vi "Cypher Driver.vi"() -> ()   [LabVIEW 2016]
uses:
  <userlib>/LevyLab/Relay Box/Type_defs/Resistor--enum.ctl
  subVIs/Driver Variables_Cypher.vi
  subVIs/Global Variables.vi
panel:
  in  "Data Queue":refnum<queue>
  in  "Amplifier Setting":dbl=-15.0
  in  "Interpolation Distance (µm)":dbl=0.1
  in  "Background Image":refnum<vi>
  in  "Inkscape File (.svg)":refnum<vi>
  in  "Run":refnum<vi>
  in  "Abort":refnum<vi>
  in  "Lithography Data":T2(array[cluster])=[{"Name"="f0", "Litho"=[{"X"=29.513355999999998, "Y"=9.417726199999999, "Speed"=5.0, "Voltage"=12.0}, {"X"=29.178072445529672, "Y"=9.536088907738542, "Speed"=5.0, "Voltage"=12.0}, {"X"=28.835439481592786, "Y"=9.643840890007512, "Speed"=5.0, "Voltage"=12.0}, {"X"=28.47974138467318, "Y"=9.7371182081142, "Speed"=5.0, "Voltage"=12.0}, {"X"=28.105262431254694, "Y"=9.812056923365887, "Speed"=5.0, "Voltage"=12.0}, {"X"=27.706286897821187, "Y"=9.864793097069871, "Speed"=5.0, "Voltage"=12.0}, {"X"=27.277099060856493, "Y"=9.891462790533431, "Speed"=5.0, "Voltage"=12.0}, {"X"=26.811983196844476, "Y"=9.88820206506386, "Speed"=5.0, "Voltage"=12.0}, {"X"=26.305223582268965, "Y"=9.851146981968443, "Speed"=5.0, "Voltage"=12.0}, {"X"=25.751104493613816, "Y"=9.776433602554466, "Speed"=5.0, "Voltage"=12.0}, {"X"=25.14391020736288, "Y"=9.660197988129223, "Speed"=5.0, "Voltage"=12.0}, {"X"=24.477925, "Y"=9.498576199999999, "Speed"=5.0, "Voltage"=12.0}, {"X"=24.477925, "Y"=9.498576199999999, "Speed"=5.0, "Voltage"=12.0}, {"X"=25.11834108313298, "Y"=9.668960284590531, "Speed"=5.0, "Voltage"=12.0}, {"X"=25.70468663448534, "Y"=9.797549343831701, "Speed"=5.0, "Voltage"=12.0}, {"X"=26.242539884259948, "Y"=9.887743940473326, "Speed"=5.0, "Voltage"=12.0}, {"X"=26.737479062659652, "Y"=9.942944637265212, "Speed"=5.0, "Voltage"=12.0}, {"X"=27.195082399887298, "Y"=9.966551996957172, "Speed"=5.0, "Voltage"=12.0}, {"X"=27.620928126145756, "Y"=9.961966582299022, "Speed"=5.0, "Voltage"=12.0}, {"X"=28.020594471637867, "Y"=9.932588956040568, "Speed"=5.0, "Voltage"=12.0}, {"X"=28.399659666566492, "Y"=9.881819680931631, "Speed"=5.0, "Voltage"=12.0}, {"X"=28.763701941134485, "Y"=9.813059319722012, "Speed"=5.0, "Voltage"=12.0}, {"X"=29.1182995255447, "Y"=9.729708435161532, "Speed"=5.0, "Voltage"=12.0}, {"X"=29.469030649999997, "Y"=9.635167589999998, "Speed"=5.0, "Voltage"=12.0}, {"X"=29.4247053, "Y"=9.85260898, "Speed"=5.0, "Voltage"=12.0}, {"X"=29.058526605559724, "Y"=9.923327962584523, "Speed"=5.0, "Voltage"=12.0}, {"X"=28.69196440067618, "Y"=9.982277749436513, "Speed"=5.0, "Voltage"=12.0}, {"X"=28.319577948459806, "Y"=10.02652115374906, "Speed"=5.0, "Voltage"=12.0}, {"X"=27.935926512021034, "Y"=10.053120988715248, "Speed"=5.0, "Voltage"=12.0}, {"X"=27.535569354470322, "Y"=10.059140067528173, "Speed"=5.0, "Voltage"=12.0}, {"X"=27.113065738918102, "Y"=10.041641203380916, "Speed"=5.0, "Voltage"=12.0}, {"X"=26.662974928474828, "Y"=9.997687209466564, "Speed"=5.0, "Voltage"=12.0}, {"X"=26.179856186250937, "Y"=9.92434089897821, "Speed"=5.0, "Voltage"=12.0}, {"X"=25.658268775356866, "Y"=9.818665085108938, "Speed"=5.0, "Voltage"=12.0}, {"X"=25.092771958903075, "Y"=9.677722581051837, "Speed"=5.0, "Voltage"=12.0}, {"X"=24.477924999999995, "Y"=9.498576199999999, "Speed"=5.0, "Voltage"=12.0}, {"X"=24.477925, "Y"=9.498576199999999, "Speed"=5.0, "Voltage"=12.0}, {"X"=25.067202834673175, "Y"=9.686484877513145, "Speed"=5.0, "Voltage"=12.0}, {"X"=25.61185091622839, "Y"=9.839780826386171, "Speed"=5.0, "Voltage"=12.0}, {"X"=26.11717248824192, "Y"=9.960937857483094, "Speed"=5.0, "Voltage"=12.0}, {"X"=26.588470794290004, "Y"=10.052429781667916, "Speed"=5.0, "Voltage"=12.0}, {"X"=27.031049077948904, "Y"=10.116730409804656, "Speed"=5.0, "Voltage"=12.0}, {"X"=27.45021058279489, "Y"=10.156313552757323, "Speed"=5.0, "Voltage"=12.0}, {"X"=27.851258552404204, "Y"=10.17365302138993, "Speed"=5.0, "Voltage"=12.0}, {"X"=28.23949623035312, "Y"=10.171222626566491, "Speed"=5.0, "Voltage"=12.0}, {"X"=28.62022686021788, "Y"=10.151496179151012, "Speed"=5.0, "Voltage"=12.0}, {"X"=28.99875368557475, "Y"=10.116947490007512, "Speed"=5.0, "Voltage"=12.0}, {"X"=29.38037995, "Y"=10.070050369999997, "Speed"=5.0, "Voltage"=12.0}, {"X"=29.336054599999997, "Y"=10.287491759999998, "Speed"=5.0, "Voltage"=12.0}, {"X"=28.938980765589776, "Y"=10.310567017430502, "Speed"=5.0, "Voltage"=12.0}, {"X"=28.548489319759575, "Y"=10.320714608865513, "Speed"=5.0, "Voltage"=12.0}, {"X"=28.159414512246432, "Y"=10.315924099383922, "Speed"=5.0, "Voltage"=12.0}, {"X"=27.766590592787374, "Y"=10.29418505406461, "Speed"=5.0, "Voltage"=12.0}, {"X"=27.364851811119458, "Y"=10.253487037986474, "Speed"=5.0, "Voltage"=12.0}, {"X"=26.94903241697971, "Y"=10.191819616228399, "Speed"=5.0, "Voltage"=12.0}, {"X"=26.513966660105183, "Y"=10.10717235386927, "Speed"=5.0, "Voltage"=12.0}, {"X"=26.054488790232902, "Y"=9.997534815987978, "Speed"=5.0, "Voltage"=12.0}, {"X"=25.565433057099916, "Y"=9.860896567663406, "Speed"=5.0, "Voltage"=12.0}, {"X"=25.04163371044327, "Y"=9.695247173974453, "Speed"=5.0, "Voltage"=12.0}, {"X"=24.477925, "Y"=9.498576199999999, "Speed"=5.0, "Voltage"=12.0}, {"X"=24.477925, "Y"=9.498576199999999, "Speed"=5.0, "Voltage"=12.0}, {"X"=25.016064586213368, "Y"=9.70400947043576, "Speed"=5.0, "Voltage"=12.0}, {"X"=25.51901519797144, "Y"=9.882012308940642, "Speed"=5.0, "Voltage"=12.0}, {"X"=25.99180509222389, "Y"=10.034131774492861, "Speed"=5.0, "Voltage"=12.0}, {"X"=26.439462525920355, "Y"=10.161914926070622, "Speed"=5.0, "Voltage"=12.0}, {"X"=26.867015756010513, "Y"=10.26690882265214, "Speed"=5.0, "Voltage"=12.0}, {"X"=27.279493039444027, "Y"=10.350660523215627, "Speed"=5.0, "Voltage"=12.0}, {"X"=27.681922633170547, "Y"=10.41471708673929, "Speed"=5.0, "Voltage"=12.0}, {"X"=28.079332794139745, "Y"=10.460625572201351, "Speed"=5.0, "Voltage"=12.0}, {"X"=28.476751779301274, "Y"=10.489933038580013, "Speed"=5.0, "Voltage"=12.0}, {"X"=28.879207845604803, "Y"=10.504186544853493, "Speed"=5.0, "Voltage"=12.0}, {"X"=29.291729249999996, "Y"=10.50493315, "Speed"=5.0, "Voltage"=12.0}, {"X"=29.2474039, "Y"=10.722374539999999, "Speed"=5.0, "Voltage"=12.0}, {"X"=28.81943492561983, "Y"=10.697806072276482, "Speed"=5.0, "Voltage"=12.0}, {"X"=28.405014238842973, "Y"=10.659151468294514, "Speed"=5.0, "Voltage"=12.0}, {"X"=27.999251076033058, "Y"=10.605327045018782, "Speed"=5.0, "Voltage"=12.0}, {"X"=27.597254673553717, "Y"=10.535249119413972, "Speed"=5.0, "Voltage"=12.0}, {"X"=27.194134267768597, "Y"=10.447834008444776, "Speed"=5.0, "Voltage"=12.0}, {"X"=26.784999095041314, "Y"=10.341998029075882, "Speed"=5.0, "Voltage"=12.0}, {"X"=26.364958391735534, "Y"=10.216657498271974, "Speed"=5.0, "Voltage"=12.0}, {"X"=25.92912139421487, "Y"=10.070728732997745, "Speed"=5.0, "Voltage"=12.0}, {"X"=25.472597338842967, "Y"=9.903128050217878, "Speed"=5.0, "Voltage"=12.0}, {"X"=24.99049546198347, "Y"=9.712771766897067, "Speed"=5.0, "Voltage"=12.0}, {"X"=24.477925, "Y"=9.498576199999999, "Speed"=5.0, "Voltage"=12.0}, {"X"=24.477925, "Y"=9.498576199999999, "Speed"=5.0, "Voltage"=12.0}, {"X"=24.964926337753568, "Y"=9.721534063358375, "Speed"=5.0, "Voltage"=12.0}, {"X"=25.42617947971449, "Y"=9.924243791495112, "Speed"=5.0, "Voltage"=12.0}, {"X"=25.866437696205857, "Y"=10.107325691502629, "Speed"=5.0, "Voltage"=12.0}, {"X"=26.29045425755071, "Y"=10.271400070473327, "Speed"=5.0, "Voltage"=12.0}, {"X"=26.70298243407212, "Y"=10.417087235499622, "Speed"=5.0, "Voltage"=12.0}, {"X"=27.108775496093163, "Y"=10.545007493673928, "Speed"=5.0, "Voltage"=12.0}, {"X"=27.512586713936884, "Y"=10.655781152088654, "Speed"=5.0, "Voltage"=12.0}, {"X"=27.91916935792637, "Y"=10.750028517836213, "Speed"=5.0, "Voltage"=12.0}, {"X"=28.333276698384672, "Y"=10.828369898009015, "Speed"=5.0, "Voltage"=12.0}, {"X"=28.759662005634855, "Y"=10.891425599699472, "Speed"=5.0, "Voltage"=12.0}, {"X"=29.203078549999997, "Y"=10.939815929999998, "Speed"=5.0, "Voltage"=12.0}, {"X"=29.1587532, "Y"=11.15725732, "Speed"=5.0, "Voltage"=12.0}, {"X"=28.69988908564988, "Y"=11.085045127122463, "Speed"=5.0, "Voltage"=12.0}, {"X"=28.261539157926368, "Y"=10.997588327723514, "Speed"=5.0, "Voltage"=12.0}, {"X"=27.839087639819684, "Y"=10.894729990653644, "Speed"=5.0, "Voltage"=12.0}, {"X"=27.427918754320057, "Y"=10.776313184763334, "Speed"=5.0, "Voltage"=12.0}, {"X"=27.023416724417732, "Y"=10.642180978903077, "Speed"=5.0, "Voltage"=12.0}, {"X"=26.620965773102924, "Y"=10.492176441923366, "Speed"=5.0, "Voltage"=12.0}, {"X"=26.215950123365886, "Y"=10.326142642674679, "Speed"=5.0, "Voltage"=12.0}, {"X"=25.803753998196843, "Y"=10.143922650007513, "Speed"=5.0, "Voltage"=12.0}, {"X"=25.379761620586017, "Y"=9.945359532772349, "Speed"=5.0, "Voltage"=12.0}, {"X"=24.939357213523664, "Y"=9.730296359819683, "Speed"=5.0, "Voltage"=12.0}, {"X"=24.477925, "Y"=9.498576199999999, "Speed"=5.0, "Voltage"=12.0}, {"X"=24.477925, "Y"=9.498576199999999, "Speed"=5.0, "Voltage"=12.0}, {"X"=24.91378808929376, "Y"=9.739058656280989, "Speed"=5.0, "Voltage"=12.0}, {"X"=25.33334376145754, "Y"=9.966475274049584, "Speed"=5.0, "Voltage"=12.0}, {"X"=25.74107030018783, "Y"=10.180519608512395, "Speed"=5.0, "Voltage"=12.0}, {"X"=26.141445989181065, "Y"=10.38088521487603, "Speed"=5.0, "Voltage"=12.0}, {"X"=26.53894911213373, "Y"=10.567265648347107, "Speed"=5.0, "Voltage"=12.0}, {"X"=26.938057952742298, "Y"=10.73935446413223, "Speed"=5.0, "Voltage"=12.0}, {"X"=27.343250794703227, "Y"=10.896845217438013, "Speed"=5.0, "Voltage"=12.0}, {"X"=27.759005921712998, "Y"=11.039431463471075, "Speed"=5.0, "Voltage"=12.0}, {"X"=28.189801617468063, "Y"=11.166806757438014, "Speed"=5.0, "Voltage"=12.0}, {"X"=28.64011616566491, "Y"=11.278664654545453, "Speed"=5.0, "Voltage"=12.0}, {"X"=29.11442785, "Y"=11.37469871, "Speed"=5.0, "Voltage"=12.0}, {"X"=29.070102499999997, "Y"=11.592140099999998, "Speed"=5.0, "Voltage"=12.0}, {"X"=28.580343245679934, "Y"=11.472284181968444, "Speed"=5.0, "Voltage"=12.0}, {"X"=28.118064077009763, "Y"=11.336025187152515, "Speed"=5.0, "Voltage"=12.0}, {"X"=27.678924203606314, "Y"=11.184132936288504, "Speed"=5.0, "Voltage"=12.0}, {"X"=27.258582835086397, "Y"=11.017377250112695, "Speed"=5.0, "Voltage"=12.0}, {"X"=26.852699181066864, "Y"=10.83652794936138, "Speed"=5.0, "Voltage"=12.0}, {"X"=26.456932451164533, "Y"=10.642354854770847, "Speed"=5.0, "Voltage"=12.0}, {"X"=26.066941854996237, "Y"=10.435627787077383, "Speed"=5.0, "Voltage"=12.0}, {"X"=25.67838660217881, "Y"=10.217116567017278, "Speed"=5.0, "Voltage"=12.0}, {"X"=25.28692590232907, "Y"=9.987591015326819, "Speed"=5.0, "Voltage"=12.0}, {"X"=24.888218965063857, "Y"=9.747820952742297, "Speed"=5.0, "Voltage"=12.0}, {"X"=24.477925, "Y"=9.498576199999999, "Speed"=5.0, "Voltage"=12.0}, {"X"=24.477925, "Y"=9.498576199999999, "Speed"=5.0, "Voltage"=12.0}, {"X"=24.862649840833956, "Y"=9.756583249203604, "Speed"=5.0, "Voltage"=12.0}, {"X"=25.240508043200595, "Y"=10.008706756604054, "Speed"=5.0, "Voltage"=12.0}, {"X"=25.615702904169794, "Y"=10.253713525522164, "Speed"=5.0, "Voltage"=12.0}, {"X"=25.992437720811417, "Y"=10.490370359278735, "Speed"=5.0, "Voltage"=12.0}, {"X"=26.374915790195338, "Y"=10.717444061194591, "Speed"=5.0, "Voltage"=12.0}, {"X"=26.767340409391434, "Y"=10.933701434590532, "Speed"=5.0, "Voltage"=12.0}, {"X"=27.17391487546957, "Y"=11.137909282787376, "Speed"=5.0, "Voltage"=12.0}, {"X"=27.598842485499624, "Y"=11.328834409105935, "Speed"=5.0, "Voltage"=12.0}, {"X"=28.04632653655146, "Y"=11.505243616867016, "Speed"=5.0, "Voltage"=12.0}, {"X"=28.520570325694962, "Y"=11.665903709391433, "Speed"=5.0, "Voltage"=12.0}, {"X"=29.02577715, "Y"=11.80958149, "Speed"=5.0, "Voltage"=12.0}, {"X"=28.981451800000002, "Y"=12.02702288, "Speed"=5.0, "Voltage"=12.0}, {"X"=28.46079740570999, "Y"=11.859523236814423, "Speed"=5.0, "Voltage"=12.0}, {"X"=27.97458899609316, "Y"=11.674462046581516, "Speed"=5.0, "Voltage"=12.0}, {"X"=27.51876076739294, "Y"=11.473535881923366, "Speed"=5.0, "Voltage"=12.0}, {"X"=27.08924691585274, "Y"=11.258441315462056, "Speed"=5.0, "Voltage"=12.0}, {"X"=26.681981637716, "Y"=11.030874919819684, "Speed"=5.0, "Voltage"=12.0}, {"X"=26.292899129226143, "Y"=10.792533267618332, "Speed"=5.0, "Voltage"=12.0}, {"X"=25.917933586626592, "Y"=10.545112931480087, "Speed"=5.0, "Voltage"=12.0}, {"X"=25.55301920616078, "Y"=10.290310484027048, "Speed"=5.0, "Voltage"=12.0}, {"X"=25.19409018407212, "Y"=10.02982249788129, "Speed"=5.0, "Voltage"=12.0}, {"X"=24.837080716604056, "Y"=9.76534554566491, "Speed"=5.0, "Voltage"=12.0}, {"X"=24.477925, "Y"=9.498576199999999, "Speed"=5.0, "Voltage"=12.0}, {"X"=24.477925, "Y"=9.498576199999999, "Speed"=5.0, "Voltage"=12.0}, {"X"=24.811511592374153, "Y"=9.774107842126218, "Speed"=5.0, "Voltage"=12.0}, {"X"=25.147672324943645, "Y"=10.050938239158524, "Speed"=5.0, "Voltage"=12.0}, {"X"=25.490335508151766, "Y"=10.32690744253193, "Speed"=5.0, "Voltage"=12.0}, {"X"=25.843429452441768, "Y"=10.59985550368144, "Speed"=5.0, "Voltage"=12.0}, {"X"=26.210882468256948, "Y"=10.867622474042072, "Speed"=5.0, "Voltage"=12.0}, {"X"=26.59662286604057, "Y"=11.128048405048833, "Speed"=5.0, "Voltage"=12.0}, {"X"=27.00457895623591, "Y"=11.378973348136737, "Speed"=5.0, "Voltage"=12.0}, {"X"=27.43867904928625, "Y"=11.618237354740796, "Speed"=5.0, "Voltage"=12.0}, {"X"=27.902851455634856, "Y"=11.843680476296015, "Speed"=5.0, "Voltage"=12.0}, {"X"=28.401024485725014, "Y"=12.053142764237414, "Speed"=5.0, "Voltage"=12.0}, {"X"=28.93712645, "Y"=12.24446427, "Speed"=5.0, "Voltage"=12.0}, {"X"=28.8928011, "Y"=12.46190566, "Speed"=5.0, "Voltage"=12.0}, {"X"=28.34125156574004, "Y"=12.246762291660403, "Speed"=5.0, "Voltage"=12.0}, {"X"=27.831113915176555, "Y"=12.012898906010516, "Speed"=5.0, "Voltage"=12.0}, {"X"=27.358597331179567, "Y"=11.762938827558227, "Speed"=5.0, "Voltage"=12.0}, {"X"=26.91991099661908, "Y"=11.499505380811417, "Speed"=5.0, "Voltage"=12.0}, {"X"=26.51126409436514, "Y"=11.225221890277984, "Speed"=5.0, "Voltage"=12.0}, {"X"=26.12886580728775, "Y"=10.942711680465814, "Speed"=5.0, "Voltage"=12.0}, {"X"=25.768925318256947, "Y"=10.654598075882792, "Speed"=5.0, "Voltage"=12.0}, {"X"=25.42765181014275, "Y"=10.363504401036815, "Speed"=5.0, "Voltage"=12.0}, {"X"=25.10125446581517, "Y"=10.07205398043576, "Speed"=5.0, "Voltage"=12.0}, {"X"=24.785942468144253, "Y"=9.782870138587526, "Speed"=5.0, "Voltage"=12.0}, {"X"=24.477925, "Y"=9.498576199999999, "Speed"=5.0, "Voltage"=12.0}, {"X"=24.477925, "Y"=9.498576199999999, "Speed"=5.0, "Voltage"=12.0}, {"X"=24.76037334391435, "Y"=9.791632435048832, "Speed"=5.0, "Voltage"=12.0}, {"X"=25.0548366066867, "Y"=10.093169721712995, "Speed"=5.0, "Voltage"=12.0}, {"X"=25.364968112133734, "Y"=10.400101359541699, "Speed"=5.0, "Voltage"=12.0}, {"X"=25.694421184072123, "Y"=10.709340648084144, "Speed"=5.0, "Voltage"=12.0}, {"X"=26.046849146318557, "Y"=11.017800886889557, "Speed"=5.0, "Voltage"=12.0}, {"X"=26.425905322689704, "Y"=11.322395375507137, "Speed"=5.0, "Voltage"=12.0}, {"X"=26.83524303700225, "Y"=11.620037413486099, "Speed"=5.0, "Voltage"=12.0}, {"X"=27.27851561307288, "Y"=11.907640300375657, "Speed"=5.0, "Voltage"=12.0}, {"X"=27.75937637471825, "Y"=12.182117335725016, "Speed"=5.0, "Voltage"=12.0}, {"X"=28.281478645755065, "Y"=12.440381819083395, "Speed"=5.0, "Voltage"=12.0}, {"X"=28.848475750000002, "Y"=12.679347049999999, "Speed"=5.0, "Voltage"=12.0}, {"X"=28.8041504, "Y"=12.89678844, "Speed"=5.0, "Voltage"=12.0}, {"X"=28.221705725770093, "Y"=12.634001346506384, "Speed"=5.0, "Voltage"=12.0}, {"X"=27.68763883425995, "Y"=12.351335765439517, "Speed"=5.0, "Voltage"=12.0}, {"X"=27.198433894966193, "Y"=12.052341773193088, "Speed"=5.0, "Voltage"=12.0}, {"X"=26.75057507738542, "Y"=11.74056944616078, "Speed"=5.0, "Voltage"=12.0}, {"X"=26.34054655101427, "Y"=11.419568860736288, "Speed"=5.0, "Voltage"=12.0}, {"X"=25.964832485349362, "Y"=11.092890093313297, "Speed"=5.0, "Voltage"=12.0}, {"X"=25.6199170498873, "Y"=10.764083220285496, "Speed"=5.0, "Voltage"=12.0}, {"X"=25.302284414124717, "Y"=10.436698318046583, "Speed"=5.0, "Voltage"=12.0}, {"X"=25.008418747558224, "Y"=10.11428546299023, "Speed"=5.0, "Voltage"=12.0}, {"X"=24.73480421968445, "Y"=9.80039473151014, "Speed"=5.0, "Voltage"=12.0}, {"X"=24.477925, "Y"=9.498576199999999, "Speed"=5.0, "Voltage"=12.0}, {"X"=24.477925, "Y"=9.498576199999999, "Speed"=5.0, "Voltage"=12.0}, {"X"=24.709235095454545, "Y"=9.809157027971448, "Speed"=5.0, "Voltage"=12.0}, {"X"=24.96200088842975, "Y"=10.135401204267465, "Speed"=5.0, "Voltage"=12.0}, {"X"=25.239600716115703, "Y"=10.473295276551466, "Speed"=5.0, "Voltage"=12.0}, {"X"=25.545412915702475, "Y"=10.818825792486848, "Speed"=5.0, "Voltage"=12.0}, {"X"=25.882815824380167, "Y"=11.167979299737038, "Speed"=5.0, "Voltage"=12.0}, {"X"=26.25518777933884, "Y"=11.516742345965437, "Speed"=5.0, "Voltage"=12.0}, {"X"=26.66590711776859, "Y"=11.86110147883546, "Speed"=5.0, "Voltage"=12.0}, {"X"=27.118352176859503, "Y"=12.19704324601052, "Speed"=5.0, "Voltage"=12.0}, {"X"=27.61590129380165, "Y"=12.520554195154016, "Speed"=5.0, "Voltage"=12.0}, {"X"=28.16193280578512, "Y"=12.827620873929375, "Speed"=5.0, "Voltage"=12.0}, {"X"=28.75982505, "Y"=13.11422983, "Speed"=5.0, "Voltage"=12.0}, {"X"=28.715499700000002, "Y"=13.33167122, "Speed"=5.0, "Voltage"=12.0}, {"X"=28.10215988580015, "Y"=13.021240401352365, "Speed"=5.0, "Voltage"=12.0}, {"X"=27.544163753343344, "Y"=12.689772624868516, "Speed"=5.0, "Voltage"=12.0}, {"X"=27.03827045875282, "Y"=12.341744718827949, "Speed"=5.0, "Voltage"=12.0}, {"X"=26.58123915815176, "Y"=11.981633511510141, "Speed"=5.0, "Voltage"=12.0}, {"X"=26.169829007663406, "Y"=11.61391583119459, "Speed"=5.0, "Voltage"=12.0}, {"X"=25.80079916341097, "Y"=11.243068506160782, "Speed"=5.0, "Voltage"=12.0}, {"X"=25.47090878151765, "Y"=10.8735683646882, "Speed"=5.0, "Voltage"=12.0}, {"X"=25.17691701810669, "Y"=10.509892235056348, "Speed"=5.0, "Voltage"=12.0}, {"X"=24.915583029301274, "Y"=10.156516945544702, "Speed"=5.0, "Voltage"=12.0}, {"X"=24.68366597122464, "Y"=9.817919324432756, "Speed"=5.0, "Voltage"=12.0}, {"X"=24.477924999999995, "Y"=9.498576199999999, "Speed"=5.0, "Voltage"=12.0}, {"X"=24.477925, "Y"=9.498576199999999, "Speed"=5.0, "Voltage"=12.0}, {"X"=24.65809684699474, "Y"=9.826681620894062, "Speed"=5.0, "Voltage"=12.0}, {"X"=24.8691651701728, "Y"=10.177632686821935, "Speed"=5.0, "Voltage"=12.0}, {"X"=25.11423332009767, "Y"=10.546489193561234, "Speed"=5.0, "Voltage"=12.0}, {"X"=25.396404647332826, "Y"=10.928310936889552, "Speed"=5.0, "Voltage"=12.0}, {"X"=25.718782502441773, "Y"=11.318157712584522, "Speed"=5.0, "Voltage"=12.0}, {"X"=26.084470235987975, "Y"=11.71108931642374, "Speed"=5.0, "Voltage"=12.0}, {"X"=26.49657119853493, "Y"=12.102165544184821, "Speed"=5.0, "Voltage"=12.0}, {"X"=26.958188740646133, "Y"=12.48644619164538, "Speed"=5.0, "Voltage"=12.0}, {"X"=27.472426212885043, "Y"=12.858991054583017, "Speed"=5.0, "Voltage"=12.0}, {"X"=28.042386965815176, "Y"=13.214859928775356, "Speed"=5.0, "Voltage"=12.0}, {"X"=28.67117435, "Y"=13.549112609999998, "Speed"=5.0, "Voltage"=12.0}], "Set Resistance"=enum."1G ohm"}, {"Name"="f1", "Litho"=[], "Set Resistance"=enum."1G ohm"}, {"Name"="p0", "Litho"=[], "Set Resistance"=enum."10M ohm"}, {"Name"="p1", "Litho"=[], "Set Resistance"=enum."100k ohm"}, {"Name"="p2", "Litho"=[], "Set Resistance"=enum."10M ohm"}, {"Name"="p3", "Litho"=[], "Set Resistance"=enum."1G ohm"}, {"Name"="p4", "Litho"=[], "Set Resistance"=enum."1G ohm"}]
  in  "Display Wave":bool
  in  "PID Close":bool
  in  "Withdraw Tip When Done":bool=TRUE
  in  "Move Z Set Point":dbl=-1.3
  in  "Z Set Point":dbl=-0.05
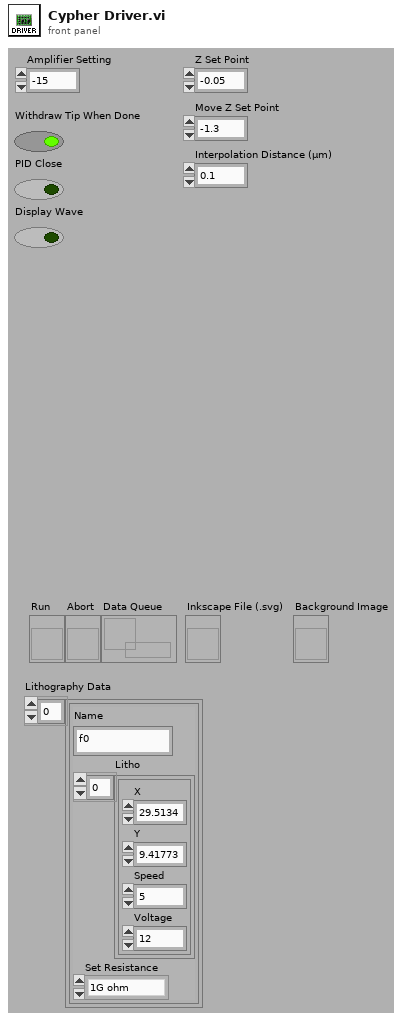
[diagram p1: front panel]
types:
  T1 = typedef "Resistor--enum.ctl" = enum16{"open", "discharge tip", "0 ohms", "100k ohm", "10M ohm", "1G ohm"}
  T2 = cluster{"Name":string, "Litho":cluster{"X":dbl, "Y":dbl, "Speed":dbl, "Voltage":dbl}[], "Set Resistance":T1}[]
  T3 = cluster{"X Offset (µm)":dbl, "Y Offset (µm)":dbl}
  T4 = cluster{"Coordinate":cluster{"X":dbl, "Y":dbl}, "Speed":dbl, "Voltage":dbl, "RGB Value":dbl, "Name":string, "Set Resistance":T1}[][]
  T5 = cluster{"Array":cluster{"Coordinate":cluster{"X":dbl, "Y":dbl}, "Speed":dbl, "Voltage":dbl, "RGB Value":dbl, "Name":string, "Set Resistance":T1}[][], "Size":cluster{"Width":dbl, "Height":dbl}, cluster{"X Offset (µm)":dbl, "Y Offset (µm)":dbl}, "Interpolation Distance (µm)":dbl, "Z Set Point":dbl, "Move Z Set Point":dbl, "PID Close":bool, "Display Wave":bool, "Run":refnum<vi>}
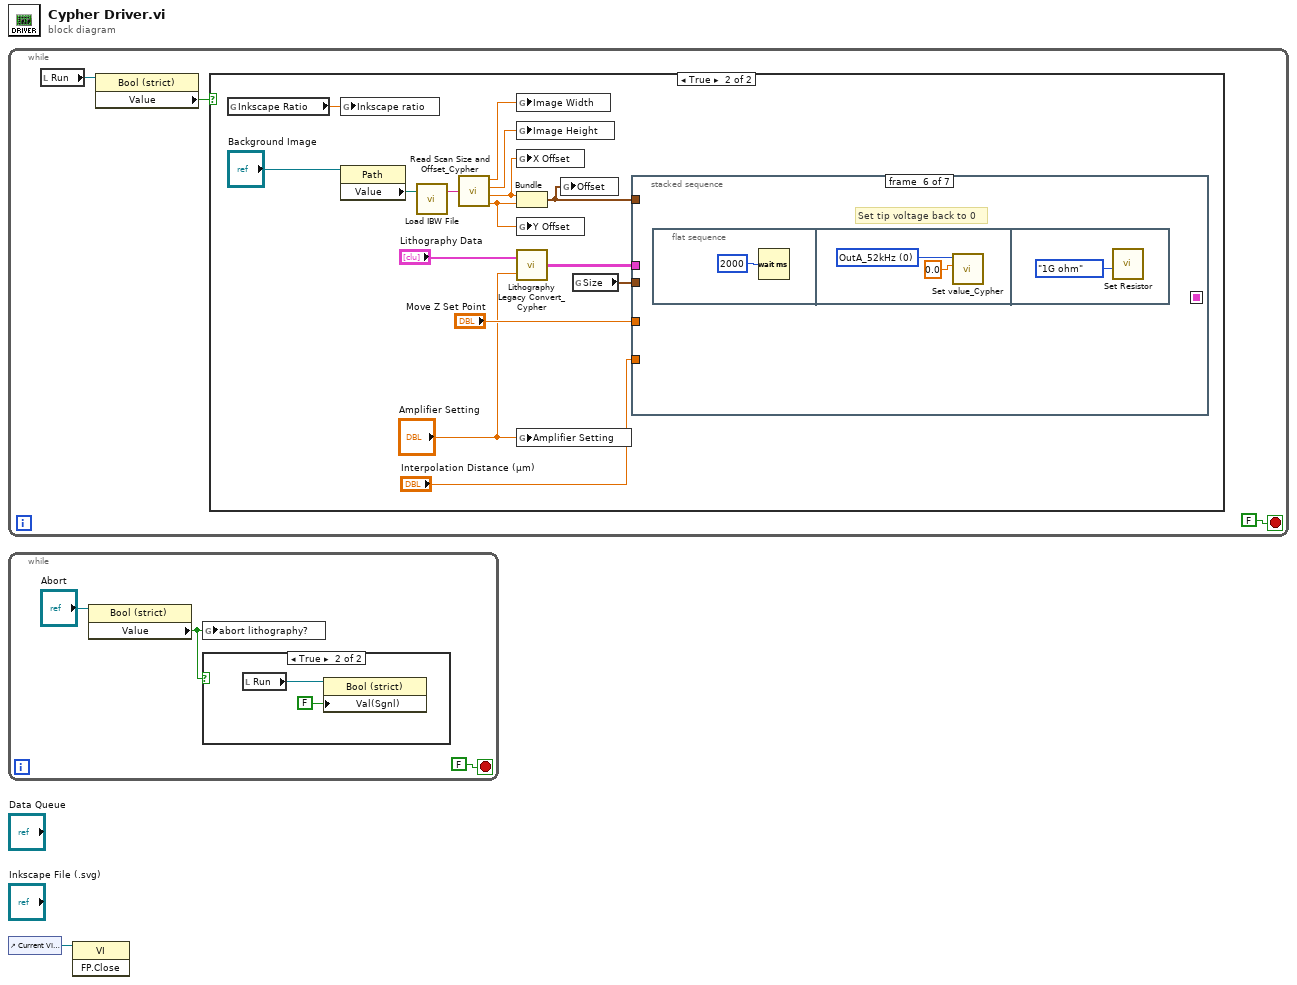
[diagram p0: block diagram]
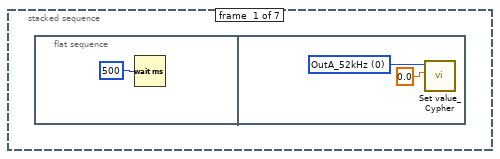
[diagram p3: hidden frame]
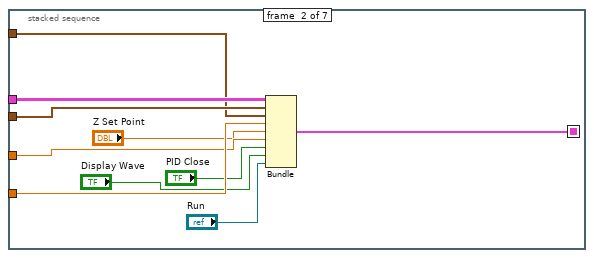
[diagram p4: hidden frame]
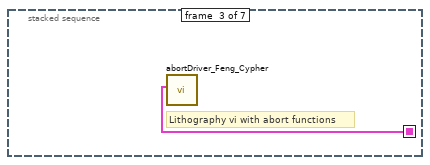
[diagram p5: hidden frame]
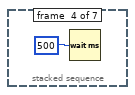
[diagram p6: hidden frame]
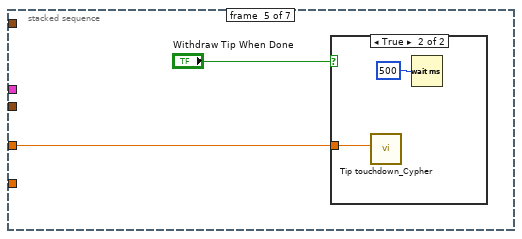
[diagram p7: hidden frame]
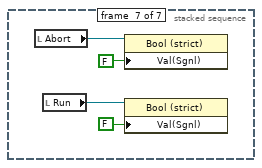
[diagram p9: hidden frame]
diagram:
  n1 = while {
    stop <- FALSE stop-if-true
    n2 = local read "Run"() -> (w3:refnum<vi>)
    n3 = property class="Bool (strict)"(reference=w3) -> ("Value"=w2:bool)  [unwired: 1 in, 2 out]
    n4 = case shown="True" w2 {
      frame False {
      }
      frame True {
        n5 = global read "Global Variables.vi" "Inkscape Ratio"() -> (w10:dbl)
        n6 = global write "Driver Variables_Cypher.vi" "Inkscape ratio"(w10) -> ()
        n7 = property class="Path"(reference="Background Image") -> ("Value"=w7:path)  [unwired: 1 in, 2 out]
        n8 = call "Load IBW File.vi"("file path (dialog if empty)"=w7) -> ("Wave Note"=w6:string)  [unwired: 1 in, 1 out]
        n9 = call "Read Scan Size and Offset_Cypher.vi"("Read in the string file"=w6) -> ("X Range (µm)"=w15:dbl, "Y Range (µm)"=w14:dbl, "X Offset (µm)"=w13:dbl, "Y Offset (µm)"=w12:dbl)  [unwired: 4 in]
        n10 = global write "Driver Variables_Cypher.vi" "Image Width"(w15) -> ()
        n11 = global write "Driver Variables_Cypher.vi" "Image Height"(w14) -> ()
        n12 = global write "Driver Variables_Cypher.vi" "X Offset"(w13) -> ()
        n13 = Bundle("X Offset (µm)"=w13, "Y Offset (µm)"=w12) -> (w11:T3)  [unwired: 1 in]
        n14 = global write "Driver Variables_Cypher.vi" "Y Offset"(w12) -> ()
        n15 = call "Lithography Legacy Convert_Cypher.vi"("Amplifier Setting"="Amplifier Setting", "Lithography Data"="Lithography Data") -> ("Array"=w9:T4)
        n16 = global write "Driver Variables_Cypher.vi" "Amplifier Setting"("Amplifier Setting") -> ()
        n17 = global write "Global Variables.vi" "Offset"(w11) -> ()
        n18 = global read "Global Variables.vi" "Size"() -> (w18:cluster{"Width":dbl, "Height":dbl})
        n19 = stacked-sequence {
          seq-local: [_ w27 _ _ _ _ _] -> [_ _ w33 _ _ _ _]
          tunnel: w9 -> [_ w32 _ _ _ _ _]
          tunnel: w18 -> [_ w31 _ _ _ _ _]
          tunnel: "Interpolation Distance (µm)" -> [_ w29 _ _ _ _ _]
          tunnel: w11 -> [_ w30 _ _ _ _ _]
          tunnel: "Move Z Set Point" -> [_ w28 _ _ w36 _ _]
          frame #0 {
            n20 = flat-sequence {
              frame #0 {
                n21 = Wait (ms)(milliseconds to wait=u32 500) -> ()  [unwired: 1 out]
              }
              frame #1 {
                w22 = u16 0 items=["OutA_52kHz", "OutB_52kHz", "OutC_78Hz", "PiezoX", "PiezoY", "PiezoZ", "DDS_Frequency1", "DDS_Frequency2", "DDS_Amplitude1", "DDS_Amplitude2", "DDS_DCOffset", "\"Setpoint%PIDSLoop.3\"", "\"Setpoint%PIDSLoop.4\"", ""] ("Output")
                n22 = call "Set value_Cypher.vi"("Value"=0.0, "Output"=w22) -> ()  [unwired: 9 in, 1 out]
              }
            }
          }
          frame #1 {
            n23 = Bundle("Array"=w32, "Size"=w31, w30, "Interpolation Distance (µm)"=w29, "Z Set Point"="Z Set Point", "Move Z Set Point"=w28, "PID Close"="PID Close", "Display Wave"="Display Wave", "Run"="Run") -> (w27:T5)  [unwired: 1 in]
          }
          frame #2 {
            # "Lithography vi with abort functions"
            n24 = call "abortDriver_Feng_Cypher.vi"("litho comm"=w33) -> ()  [unwired: 11 in]
          }
          frame #3 {
            n25 = Wait (ms)(milliseconds to wait=u32 500) -> ()  [unwired: 1 out]
          }
          frame #4 {
            n26 = case shown="True" "Withdraw Tip When Done" {
              tunnel: w36 -> [_ w37]
              frame False {
              }
              frame True {
                n27 = call "Tip touchdown_Cypher.vi"("Z SetPoint"=w37) -> ()  [unwired: 11 out]
                n28 = Wait (ms)(milliseconds to wait=u32 500) -> ()  [unwired: 1 out]
              }
            }
          }
          frame #5 {
            # "Set tip voltage back to 0"
            n29 = flat-sequence {
              frame #0 {
                n30 = Wait (ms)(milliseconds to wait=u32 2000) -> ()  [unwired: 1 out]
              }
              frame #1 {
                w41 = u16 0 items=["OutA_52kHz", "OutB_52kHz", "OutC_78Hz", "PiezoX", "PiezoY", "PiezoZ", "DDS_Frequency1", "DDS_Frequency2", "DDS_Amplitude1", "DDS_Amplitude2", "DDS_DCOffset", "\"Setpoint%PIDSLoop.3\"", "\"Setpoint%PIDSLoop.4\"", ""] ("Output")
                n31 = call "Set value_Cypher.vi"("Value"=0.0, "Output"=w41) -> ()  [unwired: 9 in, 1 out]
              }
              frame #2 {
                n32 = call <userlib>:"Set Resistor.vi"("Set Resistance"=Resistor--enum."1G ohm") -> ()  [unwired: 10 in, 1 out]
              }
            }
          }
          frame #6 {
            n33 = local read "Abort"() -> (w43:refnum<vi>)
            n34 = local read "Run"() -> (w46:refnum<vi>)
            n35 = property class="Bool (strict)"(reference=w43, "Val(Sgnl)"=FALSE ("Value (Signaling)")) -> ()  [unwired: 1 in, 2 out]
            n36 = property class="Bool (strict)"(reference=w46, "Val(Sgnl)"=FALSE ("Value (Signaling)")) -> ()  [unwired: 1 in, 2 out]
          }
        }
      }
    }
  }
  n37 = while {
    stop <- FALSE stop-if-true
    n38 = property class="Bool (strict)"(reference="Abort") -> ("Value"=w47:bool)  [unwired: 1 in, 2 out]
    n39 = global write "Driver Variables_Cypher.vi" "abort lithography?"(w47) -> ()
    n40 = case shown="True" w47 {
      frame False {
      }
      frame True {
        n41 = local read "Run"() -> (w51:refnum<vi>)
        n42 = property class="Bool (strict)"(reference=w51, "Val(Sgnl)"=FALSE ("Value (Signaling)")) -> ()  [unwired: 1 in, 2 out]
      }
    }
  }
  n43 = control-ref of="Current VI Reference"() -> (w1:refnum<vi>)
  n44 = invoke class="VI" method="FP.Close"(reference=w1) -> ()  [unwired: 2 in, 3 out]
